vi "子VI-查看某框-不显示界面.vi"(0 "框号":dbl format="%#_13g", 1 "框组":T3(array[cluster]), 2 "临界Z值":i32, 3 "反射图原始路径":path, 4 "临界面积百分比值":dbl, 5 "预先配置的灰度阈值":dbl, 6 "穿透图原始路径":path, 7 "部位信息":string[](array[string])=["", "34.500000", "32.500000", "1121", "34", "54.955926", "分层类", "不合格", ""], 12 "产品规格":cluster{"产品长度（周长）（mm）":dbl, "产品宽度（母线长）（mm）":dbl}) -> (14 "弥散类检测结果":string[][](table), 19 "分层类检测结果":string[][](table))   [LabVIEW 2018]
uses:
  <vilib>/vision/NI_Vision_Development_Module.lvlib
panel:
  in  "格式字符串 3":string="%f"
  in  "分隔符（'\\'代码显示） 2":string="\t"
  out "弥散和分层临界灰度值":i32
  out "弥散缺陷个数":i32
  out "分层缺陷个数":i32
  out "合格？ 弥散类":string="fencengThreshold"
  out "合格？分层类":string="fencengThreshold"
  out "?":T1(plugin-control)
  out "Threshold Image":T1(plugin-control)
  out "Threshold Image":T1(plugin-control)
  out "Threshold Image":T1(plugin-control)
  in  "Tab Control":T2
  out "穿透ROI":T1(plugin-control)
  out "Threshold Image":T1(plugin-control)
  out "?":T1(plugin-control)
  out "?":T1(plugin-control)
  out "Threshold Image":T1(plugin-control)
  out "Threshold Image":T1(plugin-control)
  out "弥散测量结果":dbl[][](array[numeric]) format="%.2f"
  out "面积 (pixels)":i32
  in  "格式字符串 2":string="%f"
  in  "分隔符（'\\'代码显示）":string="\t"
  out "分层测量结果":dbl[][](array[numeric]) format="%.2f"
  out "缺陷分类的临界值":sgl format="%#.3f"
  # "所选区域信息"
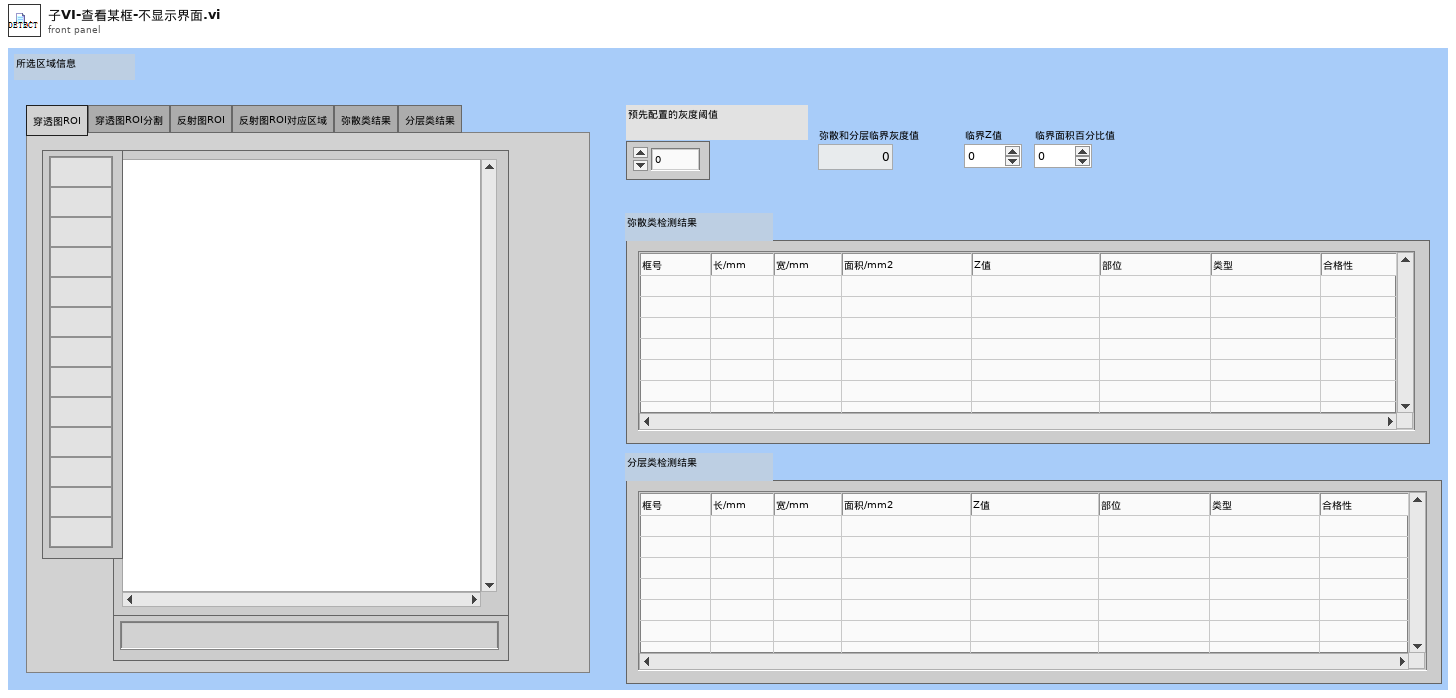
[diagram p1: front panel]
types:
  T1 = typedef "IMAQ Image.ctl" = refnum<image>
  T2 = typedef "控件 1.ctl" = enum32{"穿透图ROI", "穿透图ROI分割", "反射图ROI", "反射图ROI对应区域", "弥散类结果", "分层类结果"}
  T3 = cluster{"Global Rectangle":i32[], "Contours":cluster{"Contour Type":u32, "ROI Type":u32, "Points":i32[]}[]}[]
  T4 = typedef "Image Type" = u32
  T5 = typedef "Particle Parameters" = i32
  T6 = cluster{"Measurement Parameter":T5, "Range Lower Value":dbl, "Range Upper Value":dbl, "Range":bool, "Measurement Type":bool}[]
  T7 = cluster{"Global Rectangle":i32[], "Contours":cluster{"Contour Type":u32, "ROI Type":u32, "Points":i32[]}[]}
  T8 = cluster{"histogram":u32[], "Minimal Value":sgl, "Maximal Value":sgl, "Starting Value":sgl, "Interval Width":sgl, "Mean Value":sgl, "Standard  Variation":sgl, "Area (pixels)":i32}
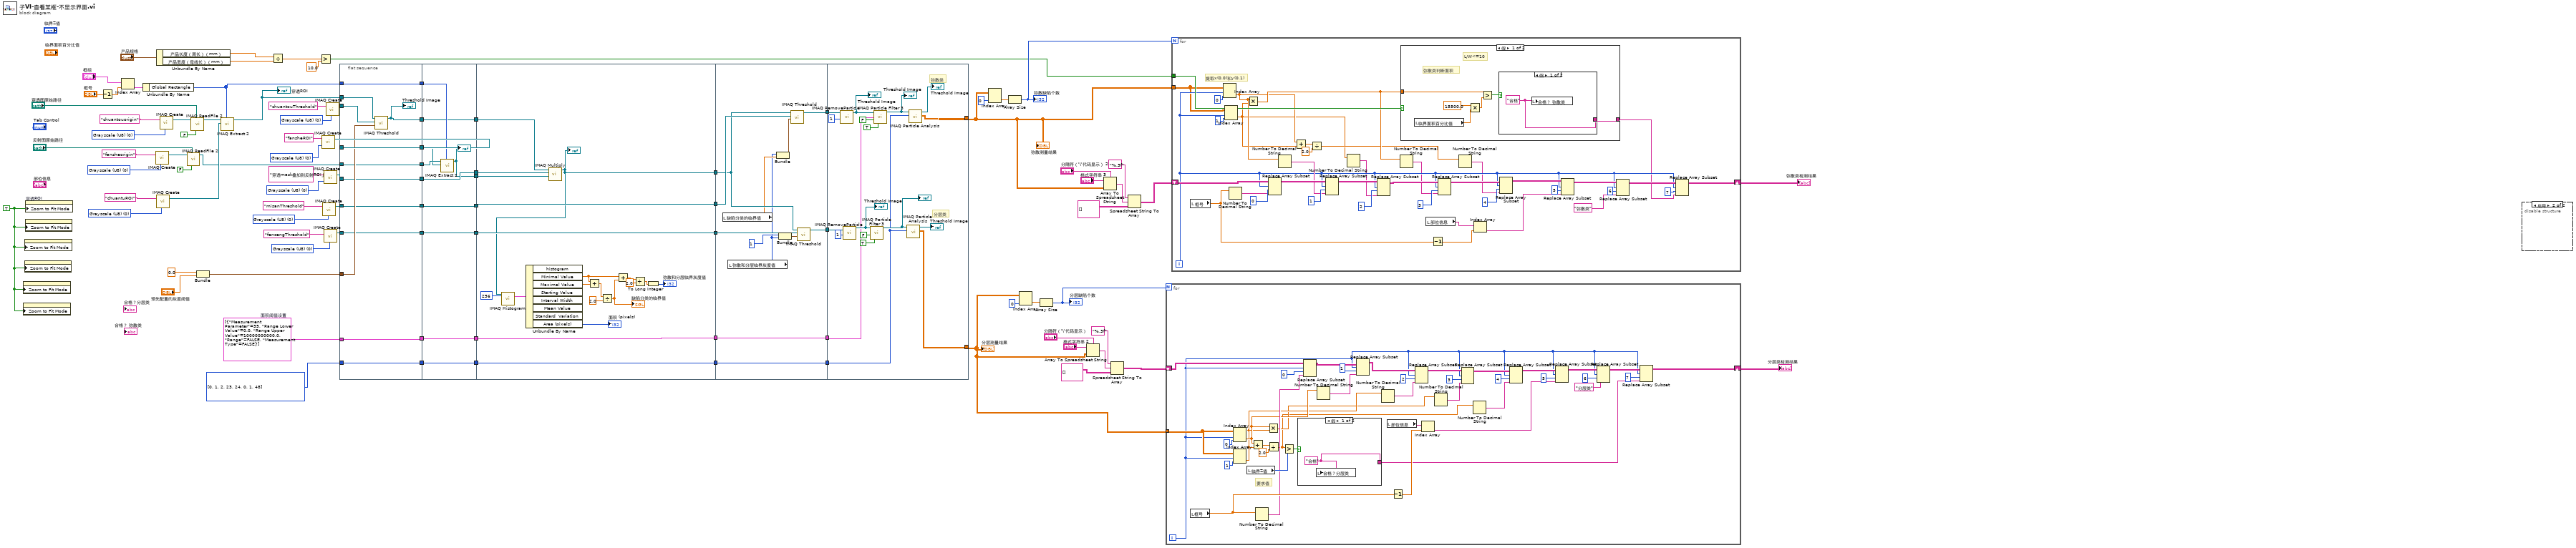
[diagram p0: block diagram]
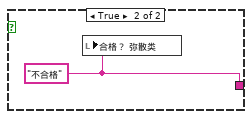
[diagram p2: hidden frame]
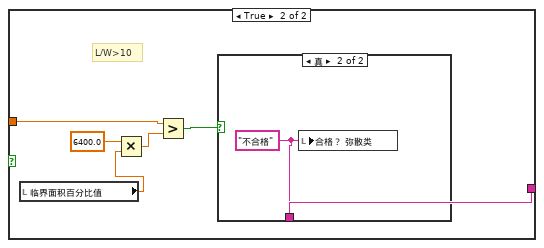
[diagram p3: hidden frame]
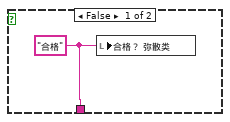
[diagram p4: hidden frame]
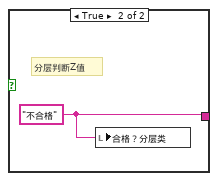
[diagram p5: hidden frame]
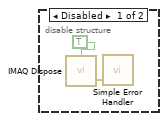
[diagram p6: hidden frame]
diagram:
  w62 = T4 0 items=["Grayscale (U8)", "Grayscale (I16)", "Grayscale (SGL)", "Complex (CSG)", "RGB (U32)", "HSL (U32)", "RGB (U64)", "Grayscale (U16)"] ("Image Type")
  w63 = T4 0 items=["Grayscale (U8)", "Grayscale (I16)", "Grayscale (SGL)", "Complex (CSG)", "RGB (U32)", "HSL (U32)", "RGB (U64)", "Grayscale (U16)"] ("Image Type")
  w64 = T4 0 items=["Grayscale (U8)", "Grayscale (I16)", "Grayscale (SGL)", "Complex (CSG)", "RGB (U32)", "HSL (U32)", "RGB (U64)", "Grayscale (U16)"] ("Image Type")
  w68 = T4 0 items=["Grayscale (U8)", "Grayscale (I16)", "Grayscale (SGL)", "Complex (CSG)", "RGB (U32)", "HSL (U32)", "RGB (U64)", "Grayscale (U16)"] ("Image Type")
  w72 = T4 0 items=["Grayscale (U8)", "Grayscale (I16)", "Grayscale (SGL)", "Complex (CSG)", "RGB (U32)", "HSL (U32)", "RGB (U64)", "Grayscale (U16)"] ("Image Type")
  w24 = i32[] [0, 1, 2, 23, 24, 0, 1, 48] items=["Bounding Rect Width", "Bounding Rect Height", "Area"] ("Pixel Measurements")
  w29 = T6 [{"Measurement Parameter"=35, "Range Lower Value"=0.0, "Range Upper Value"=10000000000.0, "Range"=FALSE, "Measurement Type"=FALSE}]  # 面积阈值设置
  w83 = T4 0 items=["Grayscale (U8)", "Grayscale (I16)", "Grayscale (SGL)", "Complex (CSG)", "RGB (U32)", "HSL (U32)", "RGB (U64)", "Grayscale (U16)"] ("Image Type")
  w56 = T4 0 items=["Grayscale (U8)", "Grayscale (I16)", "Grayscale (SGL)", "Complex (CSG)", "RGB (U32)", "HSL (U32)", "RGB (U64)", "Grayscale (U16)"] ("Image Type")
  w87 = T4 0 items=["Grayscale (U8)", "Grayscale (I16)", "Grayscale (SGL)", "Complex (CSG)", "RGB (U32)", "HSL (U32)", "RGB (U64)", "Grayscale (U16)"] ("Image Type")
  w95 = TRUE ("Zoom to Fit Mode")
  n1 = property class="ImageControl"("Zoom to Fit Mode"=w95) -> ()  [unwired: 2 in, 2 out]
  n2 = property class="ImageControl"("Zoom to Fit Mode"=w95) -> ()  [unwired: 2 in, 2 out]
  n3 = property class="ImageControl"("Zoom to Fit Mode"=w95) -> ()  [unwired: 2 in, 2 out]
  n4 = property class="ImageControl"("Zoom to Fit Mode"=w95) -> ()  [unwired: 2 in, 2 out]
  n5 = property class="ImageControl"("Zoom to Fit Mode"=w95) -> ()  [unwired: 2 in, 2 out]
  n6 = property on="穿透ROI" class="ImageControl"("Zoom to Fit Mode"=w95) -> ()  [unwired: 2 in, 2 out]
  n7 = Decrement(x="框号") -> (x-1=w89:dbl)
  n8 = Index Array(array="框组", index=w89) -> (element=w90:T7)
  n9 = Unbundle By Name(w90) -> ("Global Rectangle"=w55:i32[])
  n10 = call "IMAQ Create"("Image Name"="fansheorigin", "Image Type"=w68) -> ("New Image"=w67:T1)  [unwired: 3 in, 1 out]
  n11 = call "IMAQ Create"("Image Name"="chuantuROI", "Image Type"=w72) -> ("New Image"=w71:T1)  [unwired: 3 in, 1 out]
  n12 = Unbundle By Name("产品规格") -> ("产品长度（周长）（mm）"=w78:dbl, "产品宽度（母线长）（mm）"=w77:dbl)
  n13 = call "IMAQ Create"("Image Name"="chuantouorigin", "Image Type"=w87) -> ("New Image"=w74:T1)  [unwired: 3 in, 1 out]
  n14 = call "IMAQ ReadFile 2"("Use File Path Image Type"=FALSE, "File Path"="反射图原始路径", "Image"=w67) -> ("Image Out"=w51:T1)  [unwired: 4 in, 4 out]
  n15 = call "IMAQ ReadFile 2"("Use File Path Image Type"=FALSE, "File Path"="穿透图原始路径", "Image"=w74) -> ("Image Out"=w75:T1)  [unwired: 4 in, 4 out]
  n16 = Bundle(0.0, "预先配置的灰度阈值"="预先配置的灰度阈值") -> (w20:cluster{dbl, "预先配置的灰度阈值":dbl})  [unwired: 1 in]
  n17 = call "IMAQ Extract 2"("Optional Rectangle"=w55, "Image Dst"=w71, "Image Src"=w75) -> ("Image Dst Out"=w53:T1)  [unwired: 7 in, 1 out]
  "穿透ROI" <- w53
  n18 = Divide(x=w78, y=w77) -> (x/y=w81:dbl)
  n19 = Greater?(x=w81, y=10.0) -> (0:w4:bool)
  n20 = call "IMAQ Create"("Image Name"="fansheROI", "Image Type"=w56) -> ("New Image"=w52:T1)  [unwired: 3 in, 1 out]
  n21 = call "IMAQ Create"("Image Name"="misanThreshold", "Image Type"=w62) -> ("New Image"=w38:T1)  [unwired: 3 in, 1 out]
  n22 = call "IMAQ Create"("Image Name"="穿透mask叠加到反射ROI上", "Image Type"=w83) -> ("New Image"=w46:T1)  [unwired: 3 in, 1 out]
  n23 = call "IMAQ Create"("Image Name"="fencengThreshold", "Image Type"=w63) -> ("New Image"=w36:T1)  [unwired: 3 in, 1 out]
  n24 = call "IMAQ Create"("Image Name"="chuantouThreshold", "Image Type"=w64) -> ("New Image"=w54:T1)  [unwired: 3 in, 1 out]
  n25 = flat-sequence {
    tunnel: w55 -> [w107]
    tunnel: w54 -> [w106]
    tunnel: w53 -> [w105]
    tunnel: w20 -> [w104]
    tunnel: w52 -> [w103]
    tunnel: w51 -> [w102]
    tunnel: [w107] -> w50
    tunnel: [w103] -> w49
    tunnel: [w102] -> w48
    tunnel: [w101] -> w47
    tunnel: w46 -> [w101]
    tunnel: [w100] -> w43
    tunnel: w38 -> [w99]
    tunnel: [w99] -> w40
    tunnel: [w98] -> w37
    tunnel: w36 -> [w98]
    tunnel: [w97] -> w30
    tunnel: w29 -> [w97]
    tunnel: [w96] -> w25
    tunnel: w24 -> [w96]
    tunnel: w50 -> [w117]
    tunnel: w49 -> [w108]
    tunnel: w48 -> [w109]
    tunnel: w47 -> [w116]
    tunnel: [w116] -> w45
    tunnel: [w115] -> w44
    tunnel: w43 -> [w115]
    tunnel: [w114] -> w42
    tunnel: w40 -> [w113]
    tunnel: [w113] -> w39
    tunnel: w37 -> [w112]
    tunnel: [w112] -> w35
    tunnel: w30 -> [w111]
    tunnel: [w111] -> w28
    tunnel: w25 -> [w110]
    tunnel: [w110] -> w23
    tunnel: w45 -> [w137]
    tunnel: w44 -> [w136]
    tunnel: w42 -> [w135]
    tunnel: [w134] -> w41
    tunnel: w39 -> [w134]
    tunnel: w35 -> [w133]
    tunnel: [w133] -> w34
    tunnel: [w128] -> w33
    tunnel: w28 -> [w127]
    tunnel: [w127] -> w27
    tunnel: w23 -> [w126]
    tunnel: [w126] -> w22
    tunnel: w41 -> [w149]
    tunnel: w34 -> [w148]
    tunnel: w33 -> [w147]
    tunnel: [w146] -> w32
    tunnel: [w145] -> w31
    tunnel: w27 -> [w144]
    tunnel: [w144] -> w26
    tunnel: w22 -> [w143]
    tunnel: [w143] -> w21
    tunnel: [w153] -> w1
    tunnel: [w158] -> w14
    tunnel: w32 -> [w157]
    tunnel: w31 -> [w156]
    tunnel: w26 -> [w155]
    tunnel: w21 -> [w154]
    frame #0 {
      n26 = call "IMAQ Threshold"("Range"=w104, "Image Dst"=w106, "Image Src"=w105) -> ("Image Dst Out"=w100:T1)  [unwired: 3 in, 5 out]
      "Threshold Image" <- w100
    }
    frame #1 {
      n27 = call "IMAQ Extract 2"("Optional Rectangle"=w117, "Image Dst"=w108, "Image Src"=w109) -> ("Image Dst Out"=w114:T1)  [unwired: 7 in, 1 out]
      "?" <- w114
    }
    frame #2 {
      n28 = call "IMAQ Multiply"("Image Src A"=w136, "Image Dst"=w137, "Image Src B"=w135) -> ("Image Dst Out"=w128:T1)  [unwired: 4 in, 1 out]
      "?" <- w128
      n29 = call "IMAQ Histogram"("Number of Classes"=256, "Image"=w128) -> ("Histogram Report"=w131:T8)  [unwired: 8 in, 1 out]
      n30 = Unbundle By Name(w131) -> ("Minimal Value"=w118:sgl, "Maximal Value"=w120:sgl, "Area (pixels)"=→"面积 (pixels)":i32)  [unwired: 5 out]
      n31 = Add(x=w118, y=w120) -> (x+y=w119:sgl)
      n32 = Divide(x=w119, y=sgl 2.0) -> (x/y=w121:sgl)
      "缺陷分类的临界值" <- w121
      n33 = Add(x=w118, y=w121) -> (x+y=w125:sgl)
      n34 = Divide(x=w125, y=sgl 2.0) -> (x/y=w123:sgl)
      n35 = To Long Integer(number=w123) -> (32bit integer=→"弥散和分层临界灰度值":i32)
    }
    frame #3 {
      n36 = local read "缺陷分类的临界值"() -> (w142:sgl)
      n37 = local read "弥散和分层临界灰度值"() -> (w140:i32)
      n38 = Bundle("弥散和分层临界灰度值"=w140, "缺陷分类的临界值"=w142) -> (w141:cluster{"弥散和分层临界灰度值":i32, "缺陷分类的临界值":sgl})  [unwired: 1 in]
      n39 = Bundle(1, "弥散和分层临界灰度值"=w140) -> (w138:cluster{i32, "弥散和分层临界灰度值":i32})  [unwired: 1 in]
      n40 = call "IMAQ Threshold"("Range"=w141, "Image Dst"=w149, "Image Src"=w147) -> ("Image Dst Out"=w145:T1)  [unwired: 3 in, 5 out]
      n41 = call "IMAQ Threshold"("Range"=w138, "Image Dst"=w148, "Image Src"=w147) -> ("Image Dst Out"=w146:T1)  [unwired: 3 in, 5 out]
    }
    frame #4 {
      # "分层类"
      # "弥散类"
      n42 = call "IMAQ RemoveParticle"("Number of Erosion"=1, "Image Src"=w156) -> ("Image Dst Out"=w165:T1)  [unwired: 8 in, 1 out]
      "Threshold Image" <- w165
      n43 = call "IMAQ RemoveParticle"("Number of Erosion"=1, "Image Src"=w157) -> ("Image Dst Out"=w161:T1)  [unwired: 8 in, 1 out]
      "Threshold Image" <- w161
      n44 = call "IMAQ Particle Filter 3"("Image Src"=w161, "Keep/Remove Particles (F)"=FALSE, "Reject Border? (F)"=TRUE) -> ("Image Dst Out"=w162:T1)  [unwired: 10 in, 2 out]
      "?" <- w162
      n45 = call "IMAQ Particle Filter 3"("Image Src"=w165, "Selection Values"=w155, "Keep/Remove Particles (F)"=FALSE, "Reject Border? (F)"=TRUE) -> ("Image Dst Out"=w166:T1)  [unwired: 9 in, 2 out]
      "Threshold Image" <- w166
      n46 = call "IMAQ Particle Analysis"("Pixel Measurements"=w154, "Image"=w162) -> ("Particle Measurements (Pixels)"=w158:dbl[][], "Image Out (duplicate)"=→"Threshold Image":T1)  [unwired: 4 in, 4 out]
      n47 = call "IMAQ Particle Analysis"("Pixel Measurements"=w154, "Image"=w166) -> ("Particle Measurements (Pixels)"=w153:dbl[][], "Image Out (duplicate)"=→"Threshold Image":T1)  [unwired: 4 in, 4 out]
    }
  }
  n48 = Index Array(array=w1, index (col)=0 ("禁用的索引 (列)")) -> (element=w59:dbl[])  [unwired: 1 in]
  n49 = Array Size(array=w59) -> (size(s)=w5:i32)
  "弥散缺陷个数" <- w5
  n50 = Index Array(array=w14, index (col)=0 ("禁用的索引 (列)")) -> (element=w61:dbl[])  [unwired: 1 in]
  n51 = Array Size(array=w61) -> (size(s)=w11:i32)
  "分层缺陷个数" <- w11
  n52 = Array To Spreadsheet String(delimiter (Tab)="分隔符（'\\'代码显示）", array=w14, 3:"格式字符串 2") -> (spreadsheet string=w17:string)
  n53 = Array To Spreadsheet String(delimiter (Tab)="分隔符（'\\'代码显示） 2", array=w1, 3:"格式字符串 3") -> (spreadsheet string=w8:string)
  n54 = Spreadsheet String To Array(format string="%.3f", spreadsheet string=w17, array type (2D Dbl)=string[][] [] ("Array")) -> (array=w13:string[][])  [unwired: 1 in]
  n55 = Spreadsheet String To Array(format string="%.3f", spreadsheet string=w8, array type (2D Dbl)=string[][] [] ("Array")) -> (array=w3:string[][])  [unwired: 1 in]
  n56 = for {
    N: w11 -> [_]
    tunnel: w14 -> [w199]
    shift-right: [w177] -> w12
    shift-left: w13 -> [w188]
    i -> [w172]
    # "要求值"
    n57 = local read "框号"() -> (w197:dbl)
    n58 = Index Array(array=w199, index (row)=w172, index (col)=0 ("禁用的索引 (列)")) -> (element=w176:dbl)
    n59 = Index Array(array=w199, index (row)=w172, index (col)=1 ("禁用的索引 (列)")) -> (element=w175:dbl)
    n60 = local read "临界Z值"() -> (w205:i32)
    n61 = Add(x=w176, y=w175) -> (x+y=w206:dbl)
    n62 = Number To Decimal String(number=w197) -> (decimal integer string=w189:string)  [unwired: 1 in]
    n63 = Multiply(x=w176, y=w175) -> (x*y=w174:dbl)
    n64 = Divide(x=w206, y=2.0) -> (x/y=w171:dbl)
    n65 = Greater?(x=w171, y=w205) -> (0:w207:bool)
    n66 = case shown="假" w207 {
      tunnel: [w208 w209] -> w168
      frame False {
        w208 = "合格" ("合格？")
        n67 = local write "合格？分层类"(w208) -> ()
      }
      frame True {
        w209 = "不合格" ("合格？")
        # "分层判断Z值"
        n68 = local write "合格？分层类"(w209) -> ()
      }
    }
    n69 = Replace Array Subset(array=w188, new element=w189, index (row)=w172, index (col)=0 ("索引 (列)")) -> (w187:string[][])
    n70 = Number To Decimal String(number=w176) -> (decimal integer string=w186:string)  [unwired: 1 in]
    n71 = Replace Array Subset(array=w187, new element=w186, index (row)=w172, index (col)=1 ("索引 (列)")) -> (w184:string[][])
    n72 = Number To Decimal String(number=w175) -> (decimal integer string=w185:string)  [unwired: 1 in]
    n73 = local read "部位信息"() -> (w201:string[])
    n74 = Decrement(x=w197) -> (x-1=w200:dbl)
    n75 = Replace Array Subset(array=w184, new element=w185, index (row)=w172, index (col)=2 ("索引 (列)")) -> (w183:string[][])
    n76 = Index Array(array=w201, index=w200) -> (element=w170:string)
    n77 = Number To Decimal String(number=w174) -> (decimal integer string=w182:string)  [unwired: 1 in]
    n78 = Replace Array Subset(array=w183, new element=w182, index (row)=w172, index (col)=3 ("索引 (列)")) -> (w181:string[][])
    n79 = Number To Decimal String(number=w171) -> (decimal integer string=w173:string)  [unwired: 1 in]
    n80 = Replace Array Subset(array=w181, new element=w173, index (row)=w172, index (col)=4 ("索引 (列)")) -> (w180:string[][])
    n81 = Replace Array Subset(array=w180, new element=w170, index (row)=w172, index (col)=5 ("索引 (列)")) -> (w179:string[][])
    n82 = Replace Array Subset(array=w179, new element="分层类" ("新元素/子数组"), index (row)=w172, index (col)=6 ("索引 (列)")) -> (w178:string[][])
    n83 = Replace Array Subset(array=w178, new element=w168, index (row)=w172, index (col)=7 ("索引 (列)")) -> (w177:string[][])
  }
  "分层类检测结果" <- w12
  n84 = for {
    N: w5 -> [_]
    tunnel: w4 -> [w248]
    shift-right: [w228] -> w2
    shift-left: w3 -> [w236]
    tunnel: w1 -> [w212]
    i -> [w226]
    # "提取x(0,0)和y(0,1)"
    n85 = local read "框号"() -> (w216:dbl)
    n86 = Index Array(array=w212, index (row)=w226, index (col)=0 ("禁用的索引 (列)")) -> (element=w211:dbl)
    n87 = Index Array(array=w212, index (row)=w226, index (col)=1 ("禁用的索引 (列)")) -> (element=w210:dbl)
    n88 = Number To Decimal String(number=w216) -> (decimal integer string=w237:string)  [unwired: 1 in]
    n89 = Multiply(x=w211, y=w210) -> (x*y=w224:dbl)
    n90 = Replace Array Subset(array=w236, new element=w237, index (row)=w226, index (col)=0 ("索引 (列)")) -> (w235:string[][])
    n91 = Number To Decimal String(number=w211) -> (decimal integer string=w227:string)  [unwired: 1 in]
    n92 = Add(x=w211, y=w210) -> (x+y=w222:dbl)
    n93 = Divide(x=w222, y=2.0) -> (x/y=w220:dbl)
    n94 = Replace Array Subset(array=w235, new element=w227, index (row)=w226, index (col)=1 ("索引 (列)")) -> (w234:string[][])
    n95 = Number To Decimal String(number=w210) -> (decimal integer string=w225:string)  [unwired: 1 in]
    n96 = Replace Array Subset(array=w234, new element=w225, index (row)=w226, index (col)=2 ("索引 (列)")) -> (w233:string[][])
    n97 = Number To Decimal String(number=w224) -> (decimal integer string=w223:string)  [unwired: 1 in]
    n98 = case shown="假" w248 {
      tunnel: w224 -> [w254 w262]
      tunnel: [w252 w260] -> w213
      frame False {
        # "弥散类判断面积"
        # "L/W<=10"
        n99 = local read "临界面积百分比值"() -> (w250:dbl)
        n100 = Multiply(x=15500.0, y=w250) -> (x*y=w249:dbl)
        n101 = Greater?(x=w254, y=w249) -> (0:w253:bool)
        n102 = case shown="假" w253 {
          tunnel: [w255 w256] -> w252
          frame False {
            w255 = "合格" ("合格？")
            n103 = local write "合格？ 弥散类"(w255) -> ()
          }
          frame True {
            w256 = "不合格" ("合格？")
            n104 = local write "合格？ 弥散类"(w256) -> ()
          }
        }
      }
      frame True {
        # "L/W>10"
        n105 = local read "临界面积百分比值"() -> (w257:dbl)
        n106 = Multiply(x=6400.0, y=w257) -> (x*y=w259:dbl)
        n107 = Greater?(x=w262, y=w259) -> (0:w261:bool)
        n108 = case shown="真" w261 {
          tunnel: [w263 w264] -> w260
          frame False {
            w263 = "合格" ("合格？")
            n109 = local write "合格？ 弥散类"(w263) -> ()
          }
          frame True {
            w264 = "不合格" ("合格？")
            n110 = local write "合格？ 弥散类"(w264) -> ()
          }
        }
      }
    }
    n111 = local read "部位信息"() -> (w218:string[])
    n112 = Decrement(x=w216) -> (x-1=w217:dbl)
    n113 = Replace Array Subset(array=w233, new element=w223, index (row)=w226, index (col)=3 ("索引 (列)")) -> (w232:string[][])
    n114 = Number To Decimal String(number=w220) -> (decimal integer string=w219:string)  [unwired: 1 in]
    n115 = Index Array(array=w218, index=w217) -> (element=w215:string)
    n116 = Replace Array Subset(array=w232, new element=w219, index (row)=w226, index (col)=4 ("索引 (列)")) -> (w231:string[][])
    n117 = Replace Array Subset(array=w231, new element=w215, index (row)=w226, index (col)=5 ("索引 (列)")) -> (w230:string[][])
    n118 = Replace Array Subset(array=w230, new element="弥散类" ("新元素/子数组"), index (row)=w226, index (col)=6 ("索引 (列)")) -> (w229:string[][])
    n119 = Replace Array Subset(array=w229, new element=w213, index (row)=w226, index (col)=7 ("索引 (列)")) -> (w228:string[][])
  }
  "弥散类检测结果" <- w2
  n120 = disable-structure shown="启用" {
    frame Disabled {
      n121 = call "IMAQ Dispose"("All Images? (No)"=TRUE) -> ("error out"=w266:errorcluster)  [unwired: 5 in]
      n122 = call <vilib>:"Simple Error Handler.vi"("error in (no error)"=w266) -> ()  [unwired: 4 in, 5 out]
    }
    frame Enabled {
    }
  }
  "分层测量结果" <- w14
  "弥散测量结果" <- w1
